vi "GameConfig_FGV.vi"(7 "Mods":T2=enum."Get", 8 "error in":errorcluster) -> (0 "error out":errorcluster, 3 "Config":T1={"SpaceShip"={"Angle"=30.0, "SideLenght"=2.0, "MaxLinearVeloc"=10.0, "MaxAngularVeloc"=10.0, "LinearAceleration"=1.0, "AngularAceleration"=1.0}, "Physics"={"LinearDragFactor"=1.0, "AngularDragFactor"=1.0}, "Asteroids"={"MaxSize"=6.0, "MaxDivisions"=3, "MaxVeloc"=8.0, "MinVeloc"=1.0, "Fill"=FALSE}, "Environment"={"MaxAsteroids"=10, "TimeIncrement"=0.1, "AsterProbCreation"=0.1}, "Shots"={"MinTimeShots"=10.0, "ShotSize"=0.1, "ShotSpeed"=0.1}})   [LabVIEW 2017]
uses:
  GameConfig_mods.ctl
  GameConfig_data.ctl
  <vilib>/Utility/config.llb/NI_LVConfig.lvlib
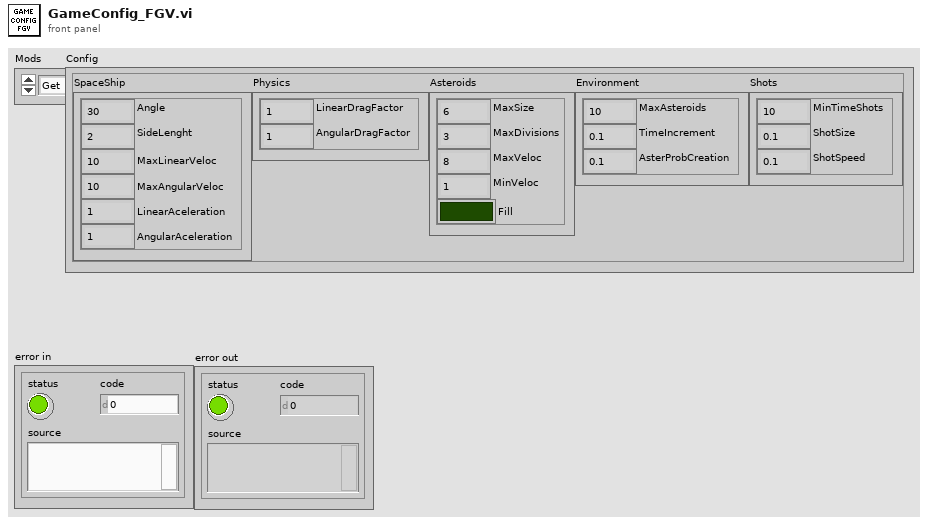
[diagram p1: front panel]
types:
  T1 = typedef "GameConfig_data.ctl" = cluster{"SpaceShip":cluster{"Angle":dbl, "SideLenght":dbl, "MaxLinearVeloc":dbl, "MaxAngularVeloc":dbl, "LinearAceleration":dbl, "AngularAceleration":dbl}, "Physics":cluster{"LinearDragFactor":dbl, "AngularDragFactor":dbl}, "Asteroids":cluster{"MaxSize":dbl, "MaxDivisions":i32, "MaxVeloc":dbl, "MinVeloc":dbl, "Fill":bool}, "Environment":cluster{"MaxAsteroids":i32, "TimeIncrement":dbl, "AsterProbCreation":dbl}, "Shots":cluster{"MinTimeShots":dbl, "ShotSize":dbl, "ShotSpeed":dbl}}
  T2 = typedef "GameConfig_mods.ctl" = enum16{"Init", "Get"}
  T3 = typedef "NI_LVConfig.lvlib/Config Data RefNum.ctl" = refnum<k1>
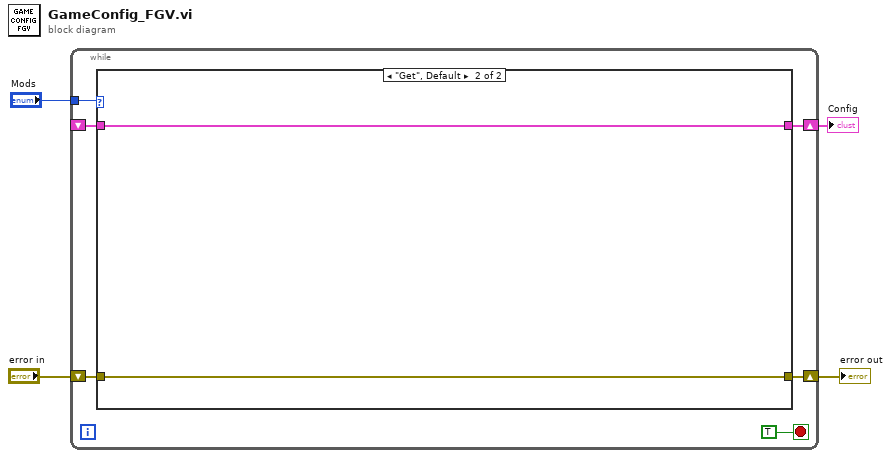
[diagram p0: block diagram]
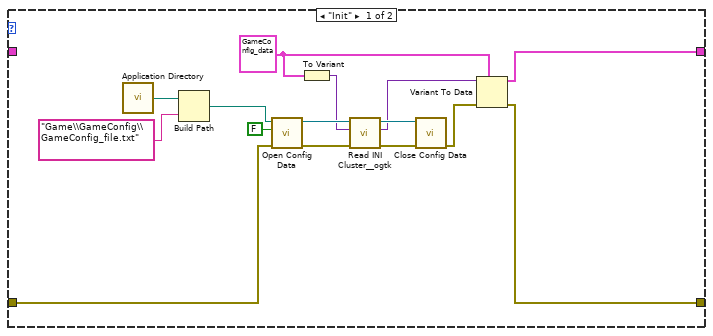
[diagram p2: hidden frame]
diagram:
  n1 = while {
    shift-right: [w7] -> w3
    shift-left: "error in" -> [w10]
    tunnel: "Mods" -> [w8]
    shift-right: [w6] -> w1
    shift-left: _ -> [w5]
    stop <- TRUE stop-if-true
    n2 = case shown="\"Get\", Default" w8 {
      tunnel: w10 -> [w21 w27]
      tunnel: [w12 w27] -> w7
      tunnel: [w11 w26] -> w6
      tunnel: w5 -> [_ w26]
      frame "Init" {
        w13 = T1 {"SpaceShip"={"Angle"=30.0, "SideLenght"=2.0, "MaxLinearVeloc"=10.0, "MaxAngularVeloc"=10.0, "LinearAceleration"=1.0, "AngularAceleration"=1.0}, "Physics"={"LinearDragFactor"=1.0, "AngularDragFactor"=1.0}, "Asteroids"={"MaxSize"=6.0, "MaxDivisions"=3, "MaxVeloc"=8.0, "MinVeloc"=1.0, "Fill"=FALSE}, "Environment"={"MaxAsteroids"=10, "TimeIncrement"=0.1, "AsterProbCreation"=0.1}, "Shots"={"MinTimeShots"=10.0, "ShotSize"=0.1, "ShotSpeed"=0.1}} ("DataCluster 2")
        n3 = call <vilib>:"Application Directory.vi"() -> ("Application Directory"=w25:path)
        n4 = Build Path(base path=w25, name or relative path="Game\\GameConfig\\GameConfig_file.txt") -> (appended path=w22:path)
        n5 = call <vilib>:"Open Config Data.vi"("error in (no error)"=w21, "create file if necessary (T)"=FALSE, "configuration file path"=w22) -> ("error out"=w20:errorcluster, "refnum"=w19:T3)  [unwired: 6 in, 1 out]
        n6 = To Variant(anything=w13) -> (Variant=w18:variant)
        n7 = call <userlib>:"Read INI Cluster__ogtk.vi"("error in (no error)"=w20, "INI Fomatted Cluster Type"=w18, "refnum"=w19) -> ("error out"=w17:errorcluster, "INI Fomatted Cluster"=w14:variant, "dup refnum"=w16:T3)  [unwired: 4 in, 2 out]
        n8 = call <vilib>:"Close Config Data.vi"("error in (no error)"=w17, "refnum"=w16) -> ("error out"=w15:errorcluster)  [unwired: 8 in, 1 out]
        n9 = Variant To Data(error in=w15, type=w13, Variant=w14) -> (data=w11:T1, error out=w12:errorcluster)
      }
      frame "Get", Default {
      }
    }
  }
  "error out" <- w3
  "Config" <- w1
